vi "CalculateExperimentValues.vi"(8 "Error In":errorcluster, 9 "Terminal Voltage (V)":dbl, 10 "Beam Current (A)":dbl, 11 "Experiment":T1={"File Path"=path "", "Operator"="", "Project"="", "Target Dose (dpa)"=0.0, "Sample"={"Name"="", "Description"="", "Molar Mass (g/mol)"=0.0, "Density (g/cm^3)"=0.0, "Irradiation Area (cm^2)"=0.0, "SRIM Damage Peak (disp * ions/cm)"=0.0}, "Beam Line"={"Type"=enum."Ion Beam Analysis", "Ion"=enum."H", "Charge State"=0, "Total Source Ion Energy (kV)"=nan}, "Runs"=[]} {"Beam Line"."Charge State" min=1}) -> (0 "Error Out":errorcluster, 1 "Total Ion Energy (MeV)":dbl, 2 "DPA Rate":dbl, 3 "Flux (ions/s * cm^2)":dbl)   [LabVIEW 2012]
uses:
  Experiment.ctl
  Sample.ctl
  BeamLine.ctl
  BeamLineType.ctl
  BeamLineIon.ctl
  ExperimentRun.ctl
  ExperimentRunTiming.ctl
  ExperimentRunDose.ctl
  ExperimentRunFluence.ctl
  ExperimentRunTotalCharge.ctl
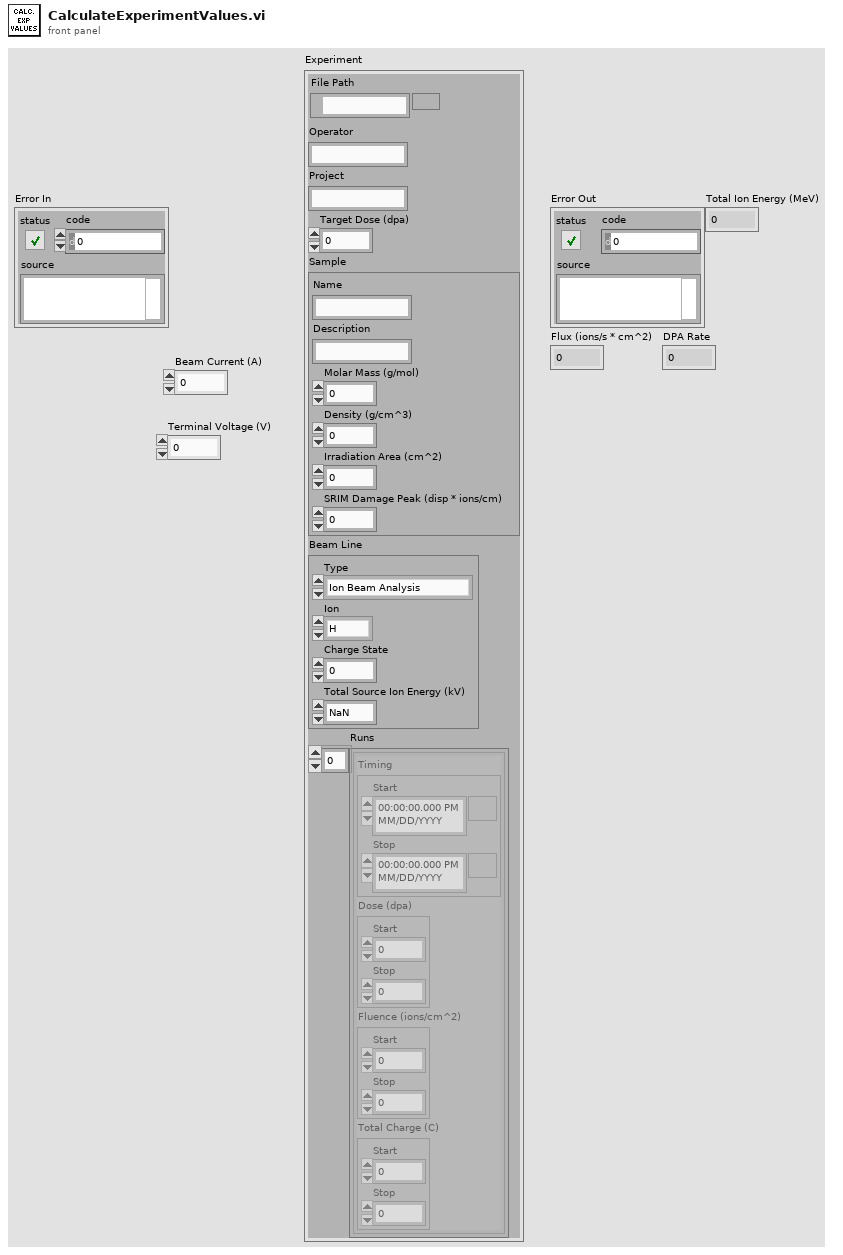
[diagram p1: front panel]
types:
  T1 = typedef "Experiment.ctl" = cluster{"File Path":path, "Operator":string, "Project":string, "Target Dose (dpa)":dbl, "Sample":T2, "Beam Line":T3, "Runs":T6[]}
  T2 = typedef "Sample.ctl" = cluster{"Name":string, "Description":string, "Molar Mass (g/mol)":dbl, "Density (g/cm^3)":dbl, "Irradiation Area (cm^2)":dbl, "SRIM Damage Peak (disp * ions/cm)":dbl}
  T3 = typedef "BeamLine.ctl" = cluster{"Type":T4, "Ion":T5, "Charge State":u8, "Total Source Ion Energy (kV)":dbl}
  T4 = typedef "BeamLineType.ctl" = enum16{"Ion Beam Analysis", "Auxiliary", "Radiation Damage"}
  T5 = typedef "BeamLineIon.ctl" = enum16{"H", "He", "C", "Fe", "Ni", "Pt", "Si", "Ag", "Au"}
  T6 = typedef "ExperimentRun.ctl" = cluster{"Timing":T7, "Dose (dpa)":T8, "Fluence (ions/cm^2)":T9, "Total Charge (C)":T10}
  T7 = typedef "ExperimentRunTiming.ctl" = cluster{"Start":timestamp, "Stop":timestamp}
  T8 = typedef "ExperimentRunDose.ctl" = cluster{"Start":dbl, "Stop":dbl}
  T9 = typedef "ExperimentRunFluence.ctl" = cluster{"Start":dbl, "Stop":dbl}
  T10 = typedef "ExperimentRunTotalCharge.ctl" = cluster{"Start":dbl, "Stop":dbl}
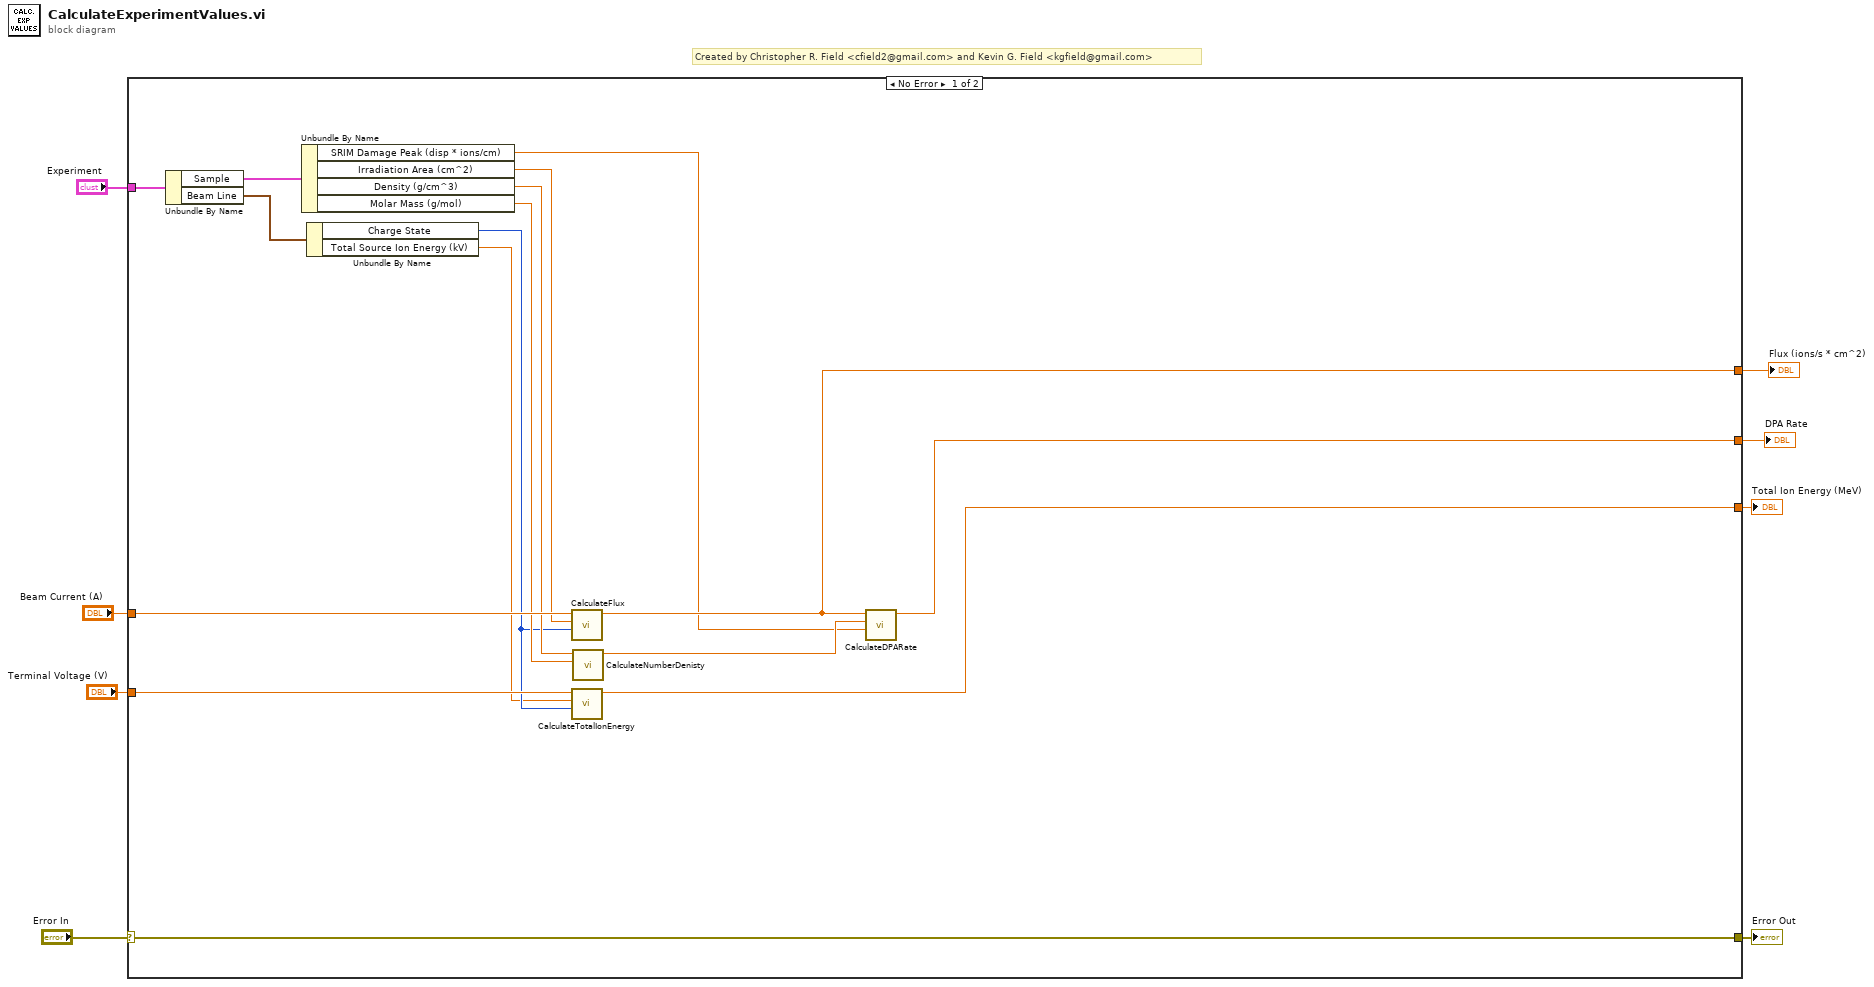
[diagram p0: block diagram]
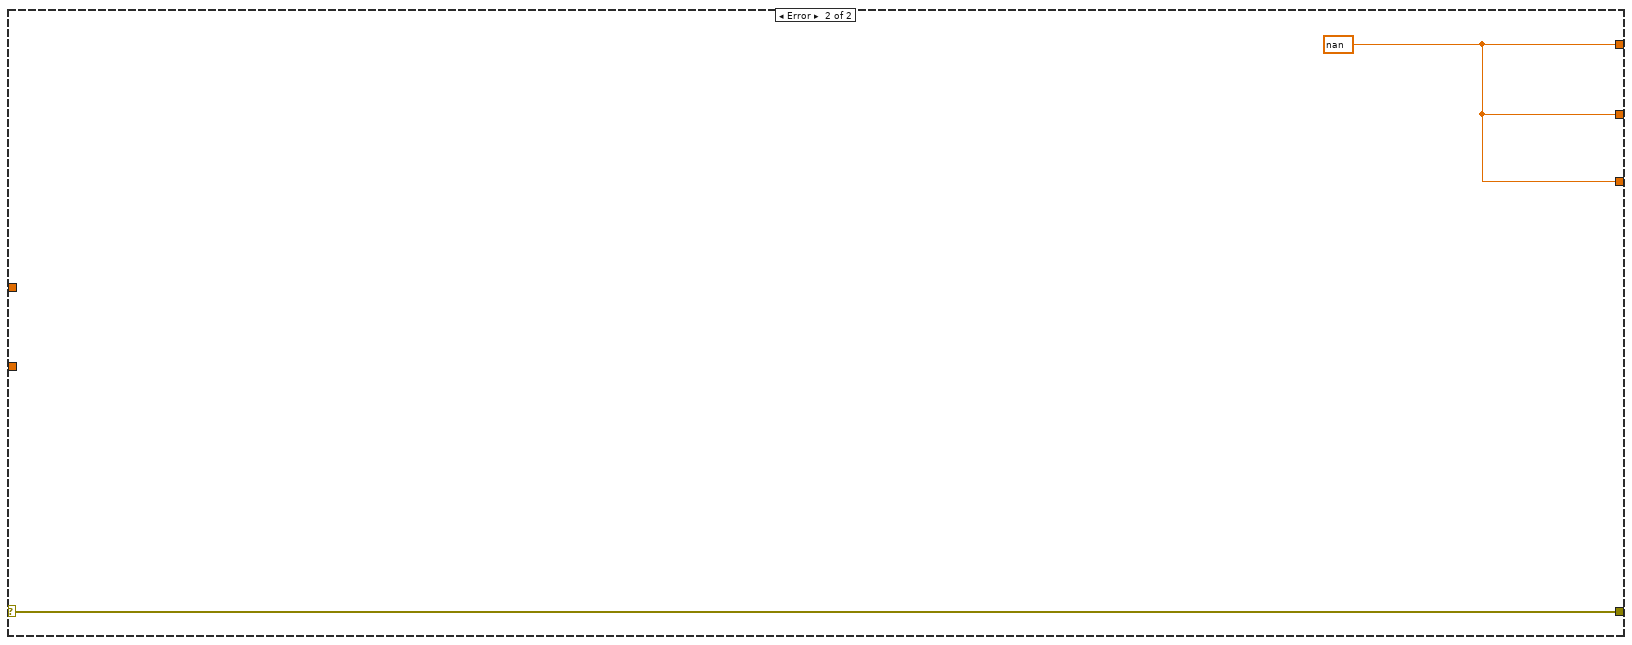
[diagram p2: hidden frame]
diagram:
  # "Created by Christopher R. Field <cfield2@gmail.com> and Kevin G. Field <kgfield@gmail.com>"
  n1 = case shown="No Error" "Error In" {
    selector: "Error In" -> [w24 w26]
    tunnel: [w24 w26] -> w7
    tunnel: "Terminal Voltage (V)" -> [w21 _]
    tunnel: "Beam Current (A)" -> [w22 _]
    tunnel: "Experiment" -> [w17 _]
    tunnel: [w20 w25] -> w3
    tunnel: [w19 w25] -> w2
    tunnel: [w18 w25] -> w1
    frame No Error {
      n2 = Unbundle By Name(w17) -> ("Sample"=w16:T2, "Beam Line"=w11:T3)
      n3 = Unbundle By Name(w16) -> ("SRIM Damage Peak (disp * ions/cm)"=w15:dbl, "Irradiation Area (cm^2)"=w14:dbl, "Density (g/cm^3)"=w13:dbl, "Molar Mass (g/mol)"=w12:dbl)
      n4 = Unbundle By Name(w11) -> ("Charge State"=w10:u8, "Total Source Ion Energy (kV)"=w9:dbl)
      n5 = call "CalculateFlux.vi"("Ion Charge State"=w10, "Irradiation Area (cm^2)"=w14, "Beam Current (A)"=w22) -> ("Flux (ions/s * cm^2)"=w20:dbl)  [unwired: 8 in]
      n6 = call "CalculateTotalIonEnergy.vi"("Ion Charge State"=w10, "Total Source Ion Energy (kV)"=w9, "Terminal Voltage (V)"=w21) -> ("Total Ion Energy (MeV)"=w18:dbl)  [unwired: 8 in]
      n7 = call "CalculateNumberDenisty.vi"("Sample Molar Mass (g/mol)"=w12, "Sample Density (g/cm^3)"=w13) -> ("Number Density (ions/cm^3)"=w23:dbl)  [unwired: 9 in]
      n8 = call "CalculateDPARate.vi"("SRIM Damage Peak (disp * ions/cm)"=w15, "Number Density (ions/cm^3)"=w23, "Flux (ions/s * cm^2)"=w20) -> ("DPA Rate"=w19:dbl)  [unwired: 8 in]
    }
    frame Error {
      w25 = nan ("Flux (ions/s * cm^2)")
    }
  }
  "Error Out" <- w7
  "Flux (ions/s * cm^2)" <- w3
  "DPA Rate" <- w2
  "Total Ion Energy (MeV)" <- w1
